vi "source_ramp_voltage.vi"(0 "Input parameters":T1={"Measurement type"=enum."Debug", "Sensor type"=enum."HPK_8in_271ch", "Identifier"="test.txt", "Open after execution?"=FALSE, "Plot after execution?"=FALSE, "Display channel"=0, "Voltage Delay (s)"=0.5, "Switch Delay (s)"=0.01, "VISA resource name source"="", "VISA resource name DMM"="", "VISA resource name LCR"="", "Compliance  Level (A)"=10.0, "Voltage Limit (V)"=1000.0, "Data storage location"="", "Scan voltages"="", "Use source as DMM?"=FALSE, "LCR signal frequenzy (Hz)"=10.0, "DMM device"=enum."Keithley2001", "Sampling number"=1, "Use env. sensors on"=enum."Sensirion sht1x/7x", "Switchboard Handle"=0, "Use Switchboard"=FALSE, "LCR signal voltage (V)"=10000.0, "Repeat"=1, "Scan voltages IV"="", "Scan voltages CV"="", "Hex pad numbers?"=FALSE, "Set measurement type"=enum."Debug", "Custom pad scan"="", "IV voltage Delay (s)"=0.5, "CV voltage Delay (s)"=0.5, "Needle measurement?"=FALSE, "Comments"="test.txt", "LCR signal frequenzy (kHz)"=10.0, "Compliance  Level (uA)"=10.0, "Open Correction Array"=array2304x3[6912 elements], "Current set voltage"=0.0, "Last set voltage"=0.0, "Current channel"=0, "Last OpenCorrection index"=-1, "Total curr/vltg every x steps"=10, "Current channel iteration"=0, "No CV corrections"=FALSE, "Mapfile"="", "Corrfile"="", "IV voltage file"=path "", "CV voltage file"=path "", "IV Switch Delay (s)"=0.01, "CV Switch Delay (s)"=0.01, "Invert polarity"=FALSE, "Set debug dirs"=FALSE, "Is n on p"=FALSE, "Source interlock?"=TRUE, "Voltage file used?"=FALSE} {"CV Switch Delay (s)" format="%#_13g"; "IV Switch Delay (s)" format="%#_13g"; "Last set voltage" format="%#_13g"; "Current set voltage" format="%#_13g"; "CV voltage Delay (s)" format="%#_13g"; "IV voltage Delay (s)" format="%#_13g"; "Voltage Limit (V)" format="%#_13g"; "Voltage Delay (s)" format="%#_13g"; "Switch Delay (s)" format="%#_13g"}, 7 "Target voltage (V)":dbl, 9 "Compliance Current (A)":dbl=0.1, 11 "error in (no error)":errorcluster, 13 "Stop":refnum<vi>) -> (4 "VISA resource name out":refnum<visa-resource-name>, 6 "Current voltage out (V)":dbl, 8 "Aborted?":bool, 15 "error out":errorcluster)   [LabVIEW 2016]
doc: "Ramps voltage up or down in specified step size."
uses:
  input_params.ctl
  <instrlib>/Keithley 24XX/Keithley 24XX.lvlib
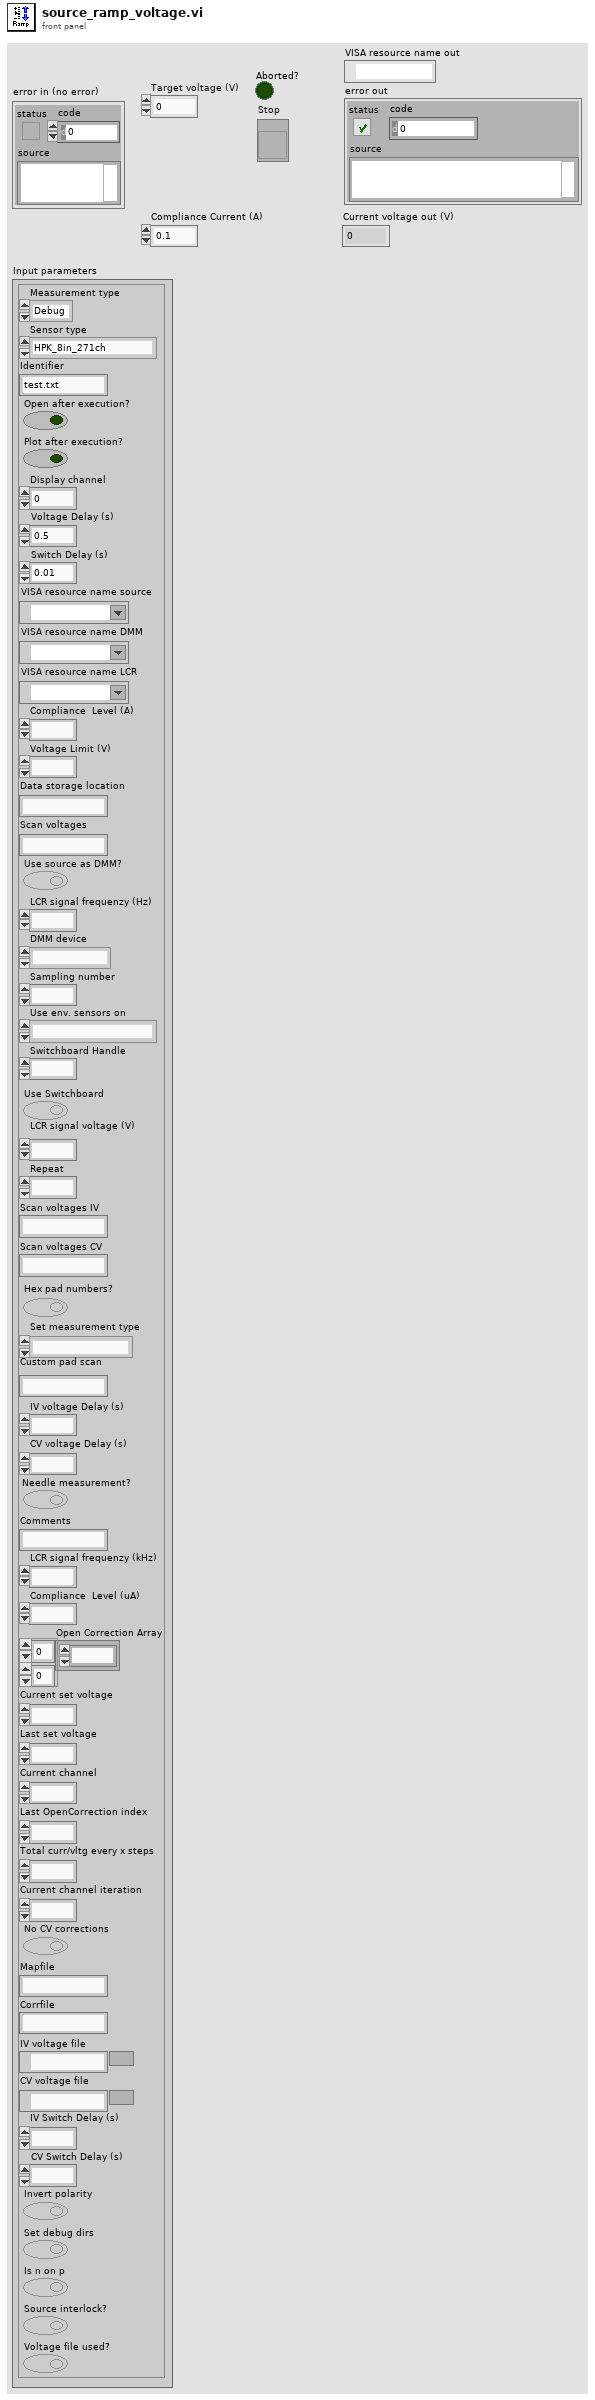
[diagram p1: front panel]
types:
  T1 = typedef "input_params.ctl" = cluster{"Measurement type":enum16{"IV", "CV", "Debug", "Test_contact"}, "Sensor type":enum16{"HPK_6in_135ch", "HPK_8in_271ch", "IFX_8in_256ch", "Diode", "HPK_6in_239ch", "Full_Matrix", ""}, "Identifier":string, "Open after execution?":bool, "Plot after execution?":bool, "Display channel":i32, "Voltage Delay (s)":dbl, "Switch Delay (s)":dbl, "VISA resource name source":refnum<visa-resource-name>, "VISA resource name DMM":refnum<visa-resource-name>, "VISA resource name LCR":refnum<visa-resource-name>, "Compliance  Level (A)":dbl, "Voltage Limit (V)":dbl, "Data storage location":string, "Scan voltages":string, "Use source as DMM?":bool, "LCR signal frequenzy (Hz)":dbl, "DMM device":enum16{"Keithley2001", "Keithley2450", "Keithley2410", "Keithley6487", "Keithley6517"}, "Sampling number":i32, "Use env. sensors on":enum16{"Sensirion sht1x/7x", "Switch Matrix", "Probecard"}, "Switchboard Handle":u32, "Use Switchboard":bool, "LCR signal voltage (V)":dbl, "Repeat":i32, "Scan voltages IV":string, "Scan voltages CV":string, "Hex pad numbers?":bool, "Set measurement type":enum16{"IV", "CV", "Debug", "Test_contact", "IV+CV"}, "Custom pad scan":string, "IV voltage Delay (s)":dbl, "CV voltage Delay (s)":dbl, "Needle measurement?":bool, "Comments":string, "LCR signal frequenzy (kHz)":dbl, "Compliance  Level (uA)":dbl, "Open Correction Array":dbl[][], "Current set voltage":dbl, "Last set voltage":dbl, "Current channel":i32, "Last OpenCorrection index":i32, "Total curr/vltg every x steps":i32, "Current channel iteration":i32, "No CV corrections":bool, "Mapfile":string, "Corrfile":string, "IV voltage file":path, "CV voltage file":path, "IV Switch Delay (s)":dbl, "CV Switch Delay (s)":dbl, "Invert polarity":bool, "Set debug dirs":bool, "Is n on p":bool, "Source interlock?":bool, "Voltage file used?":bool}
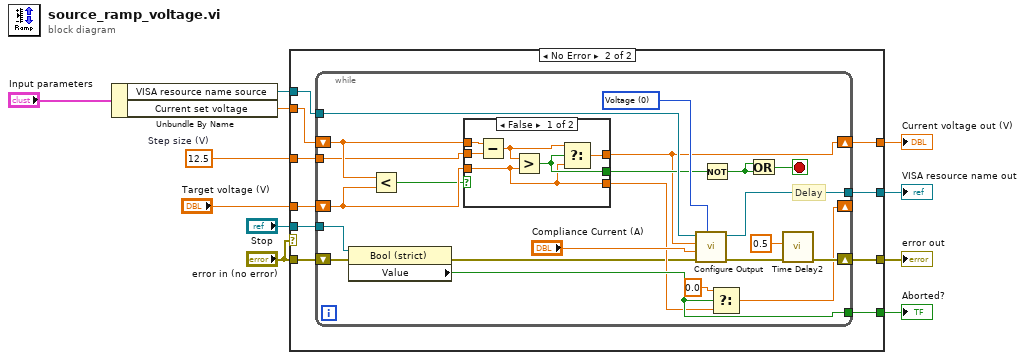
[diagram p0: block diagram]
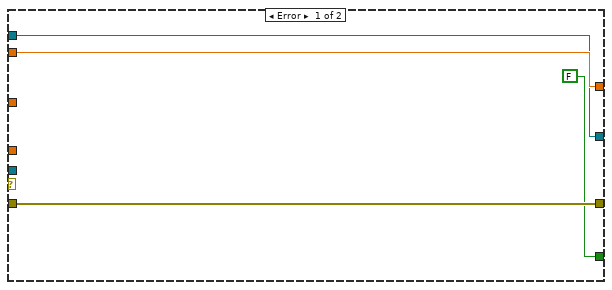
[diagram p2: hidden frame]
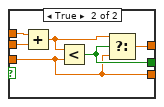
[diagram p3: hidden frame]
diagram:
  w1 = 12.5  # Step size (V)
  n1 = Unbundle By Name("Input parameters") -> ("VISA resource name source"=w3:refnum<visa-resource-name>, "Current set voltage"=w2:dbl)
  n2 = case shown="No Error" "error in (no error)" {
    tunnel: "error in (no error)" -> [w14 w25]
    tunnel: "Target voltage (V)" -> [_ w18]
    tunnel: w2 -> [w15 w19]
    tunnel: w3 -> [w13 w24]
    tunnel: [w13 w23] -> w10
    tunnel: [w14 w22] -> w9
    tunnel: [w15 w17] -> w8
    tunnel: "Stop" -> [_ w21]
    tunnel: [FALSE ("Value") w20] -> w5
    tunnel: w1 -> [_ w16]
    frame Error {
    }
    frame No Error {
      n3 = while {
        shift-right: [w34] -> w22
        shift-left: w25 -> [w28]
        shift-right: [w36] -> w17
        shift-left: w19 -> [w39]
        tunnel: w24 -> [w44]
        tunnel: [w33] -> w23
        tunnel: w21 -> [w40]
        shift-right: [w29] -> _
        shift-left: w18 -> [w38]
        tunnel: [w32] -> w20
        tunnel: w16 -> [w26]
        stop <- w43 stop-if-true
        w45 = u16 0 items=["Voltage", "Current"] ("Source Mode  (0: Voltage)")
        # "Delay"
        n4 = property class="Bool (strict)"(reference=w40, error in=w28) -> (error out=w27:errorcluster, "Value"=w32:bool)  [unwired: 1 out]
        n5 = Less?(x=w39, y=w38) -> (x < y?=w37:bool)
        n6 = case shown="False" w37 {
          tunnel: w38 -> [w48 w54]
          tunnel: w26 -> [w52 w58]
          tunnel: w39 -> [w53 w59]
          tunnel: [w50 w56] -> w36
          tunnel: [w49 w55] -> w42
          tunnel: [w48 w54] -> w30
          frame False {
            n7 = Subtract(x=w53, y=w52) -> (x-y=w51:dbl)
            n8 = Greater?(x=w51, y=w48) -> (0:w49:bool)
            n9 = Select(t=w51, s=w49, f=w48) -> (s? t:f=w50:dbl)
          }
          frame True {
            n10 = Add(x=w59, y=w58) -> (x+y=w57:dbl)
            n11 = Less?(x=w57, y=w54) -> (x < y?=w55:bool)
            n12 = Select(t=w57, s=w55, f=w54) -> (s? t:f=w56:dbl)
          }
        }
        n13 = call <instrlib>:"Configure Output.vi"("Source Mode  (0: Voltage)"=w45, "error in (no error)"=w27, "Compliance  Level (0.1)"="Compliance Current (A)", "Output Level (0)"=w36, "VISA resource name"=w44) -> ("error out"=w35:errorcluster, "VISA resource name out"=w33:refnum<visa-resource-name>)  [unwired: 5 in]
        n14 = Not(x=w42) -> (.not. x?=w41:bool)
        n15 = Select(t=0.0 ("Target voltage (V)"), s=w32, f=w30) -> (s? t:f=w29:dbl)
        n16 = Or(x=w41, y=w41) -> (x .or. y?=w43:bool)
        n17 = call "Time Delay2"("error in (no error)"=w35, "Delay Time (s)"=0.5 ("Delay (s)")) -> ("error out"=w34:errorcluster)  [unwired: 9 in]
      }
    }
  }
  "VISA resource name out" <- w10
  "error out" <- w9
  "Current voltage out (V)" <- w8
  "Aborted?" <- w5
